vi "HFRR ADV v05 new software.vi"() -> ()   [LabVIEW 2025] (continued)
                        n2289 = property on="Humidity ( %RH )" class="WFChart (strict)"("History Data"=w3352) -> ()  [unwired: 2 in, 2 out]
                        n2290 = property on="Temperature ( Deg C )" class="WFChart (strict)"("History Data"=w3352) -> ()  [unwired: 2 in, 2 out]
                        n2291 = property on="Electrical Contact Resistance ( % )" class="WFChart (strict)"("History Data"=w3352) -> ()  [unwired: 2 in, 2 out]
                        n2292 = property on="Coefficient of Friction" class="WFChart (strict)"("History Data"=w3352) -> ()  [unwired: 2 in, 2 out]
                        n2293 = property on="Frictional Force ( N )" class="WFChart (strict)"("History Data"=w3352) -> ()  [unwired: 2 in, 2 out]
                        n2294 = property on="Coefficient of Friction" class="WFChart (strict)"("History Data"=w3352) -> ()  [unwired: 2 in, 2 out]
                        n2295 = property on="Frictional Force ( N )" class="WFChart (strict)"("History Data"=w3352) -> ()  [unwired: 2 in, 2 out]
                        n2296 = property on="Electrical Contact Resistance ( % )" class="WFChart (strict)"("History Data"=w3352) -> ()  [unwired: 2 in, 2 out]
                        n2297 = property on="Humidity ( %RH )" class="WFChart (strict)"("History Data"=w3352) -> ()  [unwired: 2 in, 2 out]
                        n2298 = property on="Stroke ( mm )" class="WFChart (strict)"("History Data"=w3353) -> ()  [unwired: 2 in, 2 out]
                        n2299 = property on="Temperature ( Deg C )" class="WFChart (strict)"("History Data"=w3352) -> ()  [unwired: 2 in, 2 out]
                        n2300 = property on="Service Password Log" class="Str"("Visible"=w3354) -> ()  [unwired: 2 in, 2 out]
                        n2301 = property on="Password 3" class="Clust (strict)"("Visible"=w3354) -> ()  [unwired: 2 in, 2 out]
                      }
                    }
                    "TEST FILE NAM,E SAVED" <- TRUE ("TEST FILE NAM,E SAVED")
                  }
                }
              }
            }
          }
        }
        n2302 = case shown="True" w2661 {
          frame False {
            n2303 = local write "tfalg"(0.0 ("tfalg")) -> ()
          }
          frame True {
            n2304 = local read "tfalg"() -> (w2806:dbl)
            n2305 = Equal?(x=w2806, y=0.0) -> (x = y?=w2807:bool)
            n2306 = case shown="True" w2807 {
              frame False {
              }
              frame True {
                n2307 = local read "Total No. of Tests"() -> (w2810:dbl)
                n2308 = local write "tfalg"(1.0 ("tfalg")) -> ()
                n2309 = local write "acq 2"(FALSE ("acq 2")) -> ()
                n2310 = Wait (ms)(milliseconds to wait=u32 200) -> ()  [unwired: 1 out]
                n2311 = Increment(x=w2810) -> (x+1=w2809:dbl)
                n2312 = local write "Total No. of Tests"(w2809) -> ()
              }
            }
          }
        }
        n2313 = local write "Test \nStatus"(w2667) -> ()
        n2314 = local write "Save"(w2667) -> ()
        n2315 = local read "Main Tab"() -> (w2624:T2)
        n2316 = case shown="True" w2648 {
          tunnel: [FALSE ("RUN") TRUE ("RUN")] -> w2647
          tunnel: [_ 1] -> w2640
          frame False {
          }
          frame True {
          }
        }
        n2317 = In Range and Coerce(upper limit=w2655, x=w2628, lower limit=w2654) -> (In Range?=w2646:bool)  [unwired: 1 out]
        n2318 = In Range and Coerce(upper limit=w2652, x=w2627, lower limit=w2653) -> (In Range?=w2644:bool)  [unwired: 1 out]
        n2319 = case shown="True" w2660 {
          frame False {
            n2320 = local read "Rt 3"() -> (w2788:bool)
            n2321 = case shown="True" w2788 {
              frame False {
              }
              frame True {
                n2322 = local write "Rt 3"(FALSE ("Rt 3")) -> ()
                n2323 = local write "Json End Flg"(TRUE ("Upld AR 2")) -> ()
              }
            }
            "Rt" <- TRUE ("Rt")
            "Rt 2" <- FALSE ("Rt")
          }
          frame True {
            n2324 = local read "Rt"() -> (w2795:bool)
            n2325 = local write "Rt 2"(TRUE ("Rt 2")) -> ()
            n2326 = case shown="True" w2795 {
              frame False {
              }
              frame True {
                w2796 = TRUE ("Upld AR 2")
                n2327 = local write "Rt"(FALSE ("Rt")) -> ()
                n2328 = local write "Upld AR"(w2796) -> ()
                n2329 = local write "Json St Flg"(w2796) -> ()
              }
            }
            "Rt 3" <- TRUE ("Rt 3")
          }
        }
        n2330 = case shown="True" w2646 {
          tunnel: [FALSE ("RUN") TRUE ("RUN")] -> w2645
          tunnel: [_ 2] -> w2639
          frame False {
          }
          frame True {
          }
        }
        n2331 = case shown="True" w2644 {
          tunnel: [FALSE ("RUN") TRUE ("RUN")] -> w2643
          tunnel: [_ 3] -> w2638
          frame False {
          }
          frame True {
          }
        }
        n2332 = case shown="\"Acquire\"" w2624 {
          tunnel: w2626 -> [_ w2857]
          frame Default {
            w2856 = 0.0 ("output")
            n2333 = local write "PID-out"(w2856) -> ()
            n2334 = local write "Frequency ( Hz )"(w2856) -> ()
          }
          frame "Acquire" {
            n2335 = stacked-sequence {
              frame #0 {
                n2336 = local read "Auto Start Test"() -> (w2861:bool)
                n2337 = case shown="True" w2861 {
                  tunnel: "RUN" -> [w2882 w2885]
                  tunnel: [w2882 w2884] -> w2862
                  frame False {
                  }
                  frame True {
                    n2338 = local read "Auto Start Temp"() -> (w2883:bool)
                    n2339 = Or(x=w2885, y=w2883) -> (x .or. y?=w2884:bool)
                  }
                }
                n2340 = local read "clk"() -> (w2881:dbl)
                n2341 = local read "Save"() -> (w2877:bool)
                n2342 = Equal?(x=w2881, y=0.0) -> (x = y?=w2878:bool)
                n2343 = And(x=w2878, y=w2877) -> (x .and. y?=w2879:bool)
                n2344 = Not(x="Engage") -> (.not. x?=w2868:bool)
                n2345 = case shown="True" w2862 {
                  tunnel: [0.0 w2905] -> w2864
                  frame False {
                    (unwired) TRUE ("Visible")
                    n2346 = local read "Auto Start Test"() -> (w2889:bool)
                    n2347 = local write "Start Time"(TRUE ("Start Time")) -> ()
                    n2348 = property on="Stroke 2" class="DigNum (strict)"("Visible"=FALSE) -> ()  [unwired: 2 in, 2 out]
                    n2349 = case shown="False" w2889 {
                      frame False {
                        n2350 = property on="Heater Button" class="Bool (strict)"("DisabledEnum"=T13."Enabled" ("Disabled")) -> ()  [unwired: 2 in, 2 out]
                        n2351 = property on="Humidity" class="Bool (strict)"("DisabledEnum"=T13."Enabled" ("Disabled")) -> ()  [unwired: 2 in, 2 out]
                      }
                      frame True {
                      }
                    }
                    n2352 = case shown="False" "TestCompFlg" {
                      frame False {
                        n2353 = local read "StartFlg"() -> (w2897:bool)
                        n2354 = case shown="True" w2897 {
                          frame False {
                          }
                          frame True {
                            n2355 = flat-sequence {
                              frame #0 {
                                n2356 = local read "EVENT LOG"() -> (w2899:string)
                                n2357 = call "Event Log.vi"("Content"="Test was interrupted", "EVENT LOG"=w2899) -> ("EVENT LOG"=w2900:string)  [unwired: 8 in, 1 out]
                                n2358 = local write "EVENT LOG"(w2900) -> ()
                              }
                              frame #1 {
                                w2901 = FALSE ("StartFlg")
                                n2359 = local write "Heater Button"(w2901) -> ()
                                n2360 = local write "StartFlg"(w2901) -> ()
                                n2361 = local write "Humidity"(w2901) -> ()
                              }
                            }
                          }
                        }
                      }
                      frame True {
                      }
                    }
                    n2362 = local write "String 14"("Test will autostart once parameters reach the set value." ("String 14")) -> ()
                  }
                  frame True {
                    (unwired) FALSE ("Visible")
                    n2363 = property on="Stroke 2" class="DigNum (strict)"("Visible"=TRUE) -> ()  [unwired: 2 in, 2 out]
                    n2364 = property on="STOP 2" class="Bool (strict)"("Disabled"=u8 2) -> ()  [unwired: 2 in, 2 out]
                    n2365 = local write "String 14"(" Running....." ("String 14")) -> ()
                    n2366 = property on="Heater Button" class="Bool (strict)"("DisabledEnum"=T13."Disabled and Grayed Out" ("Disabled")) -> ()  [unwired: 2 in, 2 out]
                    n2367 = property on="Humidity" class="Bool (strict)"("DisabledEnum"=T13."Disabled and Grayed Out" ("Disabled")) -> ()  [unwired: 2 in, 2 out]
                    n2368 = case shown="True" "Start Time" {
                      selector: "Start Time" -> [_ w2917]
                      frame False {
                      }
                      frame True {
                        n2369 = Not(x=w2917) -> (.not. x?=w2916:bool)
                        n2370 = local write "Start Time"(w2916) -> ()
                        n2371 = local read "EVENT LOG"() -> (w2918:string)
                        n2372 = call "Event Log.vi"("Content"="Test in progress", "EVENT LOG"=w2918) -> ("EVENT LOG"=w2920:string)  [unwired: 8 in, 1 out]
                        n2373 = local write "EVENT LOG"(w2920) -> ()
                      }
                    }
                    n2374 = local read "Set Hz"() -> (w2914:dbl)
                    n2375 = call <vilib>:"Uniform White Noise Waveform.vi"() -> ("signal out"=w2913:waveform(dbl))  [unwired: 10 in, 1 out]
                    n2376 = Random Number (0-1)() -> (number: 0 to 1=w2904:dbl)
                    n2377 = Add(x=w2914, y=w2913) -> (x+y=w2912:waveform(dbl))
                    n2378 = Multiply(x=ext 0.05 ("y"), y=w2904) -> (x*y=w2902:ext)
                    n2379 = Multiply(x=w2912, y=w2902) -> (x*y=w2905:waveform(ext))
                    "StartFlg" <- TRUE ("StartFlg")
                  }
                }
                n2380 = case shown="True" w2879 {
                  frame False {
                  }
                  frame True {
                    n2381 = local write "clk"(10.0 ("clk")) -> ()
                    n2382 = Get Date/Time In Seconds() -> (seconds since 1Jan1904=w2923:timestamp)
                    n2383 = To Double Precision Float(number=w2923) -> (double precision float=w2921:dbl)
                    n2384 = local write "acq timer"(w2921) -> ()
                    n2385 = local write "act save time"(w2921) -> ()
                  }
                }
                n2386 = call "Elapsed Time"("Time Target (s)"="Countdown", "Reset"=w2868) -> ("Elapsed Time (s)"=w2873:dbl, "Time has Elapsed"=w2871:bool)  [unwired: 10 in, 6 out]
                "Countdown 2" <- w2873
                n2387 = Subtract(x=w2873, y=2.0) -> (x-y=w2876:dbl)
                n2388 = Less?(x=w2876, y="Countdown") -> (x < y?=w2874:bool)
                n2389 = And(x=w2874, y=w2871) -> (x .and. y?=w2870:bool)
                n2390 = case shown="True" w2870 {
                  frame False {
                  }
                  frame True {
                    (unwired) dbl[] [] ("History Data")
                    n2391 = local write "Engage"(FALSE ("Engage")) -> ()
                    n2392 = local write "RUN"(TRUE ("RUN")) -> ()
                    n2393 = local read "Humidity ( %RH )"() -> (→"Rh Before":dbl)
                  }
                }
                n2394 = Add(x=w2864, y=50.0) -> (x+y=w2860:dbl)
                n2395 = local read "Test \nStatus"() -> (w2866:bool)
                n2396 = Select(t=w2860, s=w2866, f=0.0) -> (s? t:f=w2865:dbl)
                n2397 = local write "Frequency ( Hz )"(w2865) -> ()
              }
              frame #1 {
                w2946 = 1000000.0 ("x")
                # "HC;1/0\nST;VALUE"
                # "Elapsed time\ncof\nstroke\nAir temp\nTemp\nHumidity"
                # "acq timer\n\nact save time"
                # "convert to microseconds"
                n2398 = local read "COUNT"() -> (w2929:i32)
                n2399 = local read "Rate"() -> (w2942:dbl)
                n2400 = Divide(x=w2946, y=w2942) -> (x/y=w2947:dbl)
                n2401 = Greater Or Equal?(x=w2929, y=250) -> (x >= y?=w2928:bool)
                n2402 = Get Date/Time In Seconds() -> (seconds since 1Jan1904=w2949:timestamp)
                n2403 = case shown="True" w2928 {
                  frame False {
                    n2404 = local read "COUNT"() -> (w2950:i32)
                    n2405 = Increment(x=w2950) -> (x+1=w2951:i32)
                    n2406 = local write "COUNT"(w2951) -> ()
                  }
                  frame True {
                    n2407 = local write "COUNT"(0 ("COUNT")) -> ()
                  }
                }
                n2408 = local read "Samplingtime 2"() -> (w2927:dbl)
                n2409 = local read "act save time"() -> (w2944:dbl)
                n2410 = Divide(x=w2947, y=w2946) -> (x/y=w2945:dbl)
                n2411 = To Double Precision Float(number=w2949) -> (double precision float=w2938:dbl)
                n2412 = Add(x=w2944, y=w2927) -> (x+y=w2943:dbl)
                n2413 = local read "acq timer"() -> (w2948:dbl)
                n2414 = local read "COUNT"() -> (w2931:i32)
                n2415 = Greater Or Equal?(x=w2938, y=w2943) -> (x >= y?=w2926:bool)
                n2416 = Multiply(x=w2945, y=w2931) -> (x*y=w2937:dbl)
                n2417 = Subtract(x=w2938, y=w2948) -> (x-y=w2940:dbl)
                n2418 = local read "Save"() -> (w2941:bool)
                n2419 = Add(x=w2940, y=w2937) -> (x+y=w2924:dbl)
                "Elapsed time 3" <- w2924
                n2420 = And(x=w2926, y=w2941) -> (x .and. y?=w2939:bool)
                n2421 = Divide(x=w2924, y=60.0) -> (x/y=w2935:dbl)
                n2422 = local read "Test \nStatus"() -> (w2925:bool)
                n2423 = local read "clk"() -> (w2932:dbl)
                n2424 = Equal?(x=w2932, y=10.0) -> (x = y?=w2934:bool)
                n2425 = case shown="True" w2939 {
                  tunnel: w2938 -> [_ w3060]
                  tunnel: [FALSE ("Boolean 2") TRUE ("Boolean 2")] -> _
                  frame False {
                  }
                  frame True {
                    w3014 = ";" ("Substring")
                    # "Pid out/\nFreq response value"
                    n2426 = local write "act save time"(w3060) -> ()
                    n2427 = local read "FILE"() -> (w3008:string)
                    n2428 = call "file check.vi"("file name in"=w3008) -> ("error out"=w3011:errorcluster, "file name out"=w3006:string)  [unwired: 9 in]
                    n2429 = call "FILE PATH CREATION.vi"("error in"=w3011, "FILE NAME :"=w3006) -> ("FILE OUT"=w3009:path)  [unwired: 8 in, 1 out]
                    n2430 = Concatenate Strings(w3006, ".dgf" ("Substring")) -> (w3010:string)
                    n2431 = local read "FF 2"() -> (→"Frictional Force ( N )" →"Frictional Force ( N )":dbl)
                    n2432 = Build Path(base path=w3009, name or relative path=w3010) -> (appended path=w3005:path)
                    n2433 = local read "COF 2"() -> (w3019:dbl)
                    "cof" <- w3019
                    "Coefficient of Friction" <- w3019
                    "COF 4" <- w3019
                    "Coefficient of Friction" <- w3019
                    n2434 = local read "LVDT STROKE"() -> (w3003:dbl)
                    n2435 = local read "Add up Stroke"() -> (w3001:dbl)
                    n2436 = local read "TEMP"() -> (w3022:dbl)
                    "Temp" <- w3022
                    "Temperature ( Deg C )" <- w3022
                    n2437 = local read "Humidity ( %RH )"() -> (w3021:dbl)
                    "Humidity ( %RH )" <- w3021
                    "Humidity ( %RH )" <- w3021
                    n2438 = local read "Frequency ( Hz )"() -> (w3028:dbl)
                    n2439 = local read "Elapsed time"() -> (w3053:dbl)
                    n2440 = local read "AIR TEMP"() -> (w3026:dbl)
                    n2441 = local read "PID-out"() -> (w3031:dbl)
                    n2442 = Subtract(x=w3003, y=w3001) -> (x-y=w3002:dbl)
                    n2443 = Absolute Value(x=w3002) -> (abs(x)=w3000:dbl)
                    n2444 = local write "Temperature ( Deg C )"(w3022) -> ()
                    n2445 = Number To Fractional String(number=w3000, width (-)=i16 9 ("precision (6)"), precision (6)=i16 6) -> (F-format string=w3046:string)  [unwired: 1 in]
                    n2446 = Number To Fractional String(number=w3026, width (-)=i16 9 ("precision (6)"), precision (6)=i16 3) -> (F-format string=w3045:string)  [unwired: 1 in]
                    n2447 = Number To Fractional String(number=w3022, width (-)=i16 9 ("precision (6)"), precision (6)=i16 3) -> (F-format string=w3042:string)  [unwired: 1 in]
                    n2448 = Number To Fractional String(number=w3021, width (-)=i16 9 ("precision (6)"), precision (6)=i16 3) -> (F-format string=w3039:string)  [unwired: 1 in]
                    n2449 = Number To Fractional String(number=0.0, width (-)=i16 9 ("precision (6)"), precision (6)=i16 3) -> (F-format string=w3036:string)  [unwired: 1 in]
                    n2450 = Number To Fractional String(number=w3031, width (-)=i16 9 ("precision (6)"), precision (6)=i16 3) -> (F-format string=w3032:string)  [unwired: 1 in]
                    n2451 = Number To Fractional String(number=w3028, width (-)=i16 9 ("precision (6)"), precision (6)=i16 3) -> (F-format string=w3027:string)  [unwired: 1 in]
                    n2452 = Number To Fractional String(number=w3019, width (-)=i16 9 ("precision (6)"), precision (6)=i16 6) -> (F-format string=w3054:string)  [unwired: 1 in]
                    n2453 = Number To Fractional String(number=w3053, width (-)=i16 14 ("precision (6)"), precision (6)=i16 3) -> (F-format string=w3055:string)  [unwired: 1 in]
                    n2454 = Bundle("y"=1.02, w3000, "y"=0.98) -> (w3020:cluster{"y":dbl, dbl, "y":dbl})  [unwired: 1 in]
                    n2455 = Number To Fractional String(number="Ambient Humidity :", width (-)=i16 9 ("precision (6)"), precision (6)=i16 6) -> (F-format string=w3012:string)  [unwired: 1 in]
                    n2456 = local read "RUN"() -> (w3018:bool)
                    n2457 = case shown="True" w3018 {
                      tunnel: w3020 -> [_ w3065]
                      tunnel: w3000 -> [_ w3064]
                      tunnel: w3000 -> [_ w3062]
                      tunnel: w3000 -> [_ w3063]
                      frame False {
                      }
                      frame True {
                        "Stroke ( mm )" <- w3065
                        "Stroke ( mm )" <- w3065
                        "Stroke 4" <- w3064
                        "Stroke 3" <- w3062
                        "Stroke 2" <- w3063
                        "measured_stroke" <- w3062
                      }
                    }
                    n2458 = Concatenate Strings(w3055, w3014, w3054, w3014, w3046, w3014, w3045, w3014, w3042, w3014, w3039, w3014, w3036, w3014, w3032, w3014, w3027, w3014, w3012, "\r") -> (w3052:string)
                    n2459 = call <vilib>:"Write Characters To File.vi"("append to file? (new file:F)"=TRUE, "character string"=w3052, "file path (dialog if empty)"=w3005) -> ()  [unwired: 2 in, 1 out]
                    "refresh flag" <- TRUE ("refresh flag")
                  }
                }
                n2460 = case shown="True" w2925 {
                  tunnel: w2935 -> [_ w2961]
                  tunnel: w2940 -> [_ w2971]
                  tunnel: [0.0 w2967] -> _
                  tunnel: w2934 -> [_ w2966]
                  tunnel: [0.0 w2965] -> _
                  tunnel: w2924 -> [_ w2965]
                  tunnel: w2938 -> [w2954 _]
                  frame False {
                    n2461 = local write "acq timer"(w2954) -> ()
                    n2462 = local write "Test Duration Status"(0.0 ("Test Duration Status")) -> ()
                  }
                  frame True {
                    n2463 = local read "Set Hz"() -> (w2968:dbl)
                    n2464 = local write "Elapsed time"(w2961) -> ()
                    n2465 = local read "test time"() -> (w2960:dbl)
                    n2466 = Multiply(x=w2971, y=w2968) -> (x*y=w2970:dbl)
                    n2467 = case shown="False" w2966 {
                      tunnel: w2970 -> [w2972 _]
                      tunnel: [w2972 1.0] -> w2967
                      frame False {
                        n2468 = local write "Cycles elapsed"(w2972) -> ()
                      }
                      frame True {
                      }
                    }
                    n2469 = Greater?(x=w2961, y=w2960) -> (0:w2969:bool)
                    n2470 = Subtract(x=w2960, y=w2961) -> (x-y=w2959:dbl)
                    "time" <- w2959
                    n2471 = Multiply(x=w2959, y=60.0) -> (x*y=w2958:dbl)
                    n2472 = local write "Time Remaining"(w2958) -> ()
                    n2473 = local write "Remaining Time"(w2958) -> ()
                    n2474 = case shown="True" w2969 {
                      frame False {
                      }
                      frame True {
                        n2475 = stacked-sequence {
                          frame #0 {
                            w2975 = T13."Enabled" ("Disabled")
                            w2974 = FALSE ("TEST FILE NAM,E SAVED")
                            w2978 = "" ("FILE")
                            w2979 = TRUE ("Visible")
                            n2476 = local write "Humidity"(FALSE ("Humidity")) -> ()
                            n2477 = local write "RUN"(FALSE ("OK Button 2")) -> ()
                            n2478 = local write "Heater Button"(FALSE ("Heater Button")) -> ()
                            n2479 = local write "Auto Start Test"(FALSE ("Auto Start Test")) -> ()
                            n2480 = local write "TestCompFlg"(TRUE ("StpFlg")) -> ()
                            n2481 = local read "Humidity ( %RH )"() -> (→"Rh After":dbl)
                            n2482 = property on="STOP 2" class="Bool (strict)"("Disabled"=u8 0) -> ()  [unwired: 2 in, 2 out]
                            n2483 = local read "EVENT LOG"() -> (w2984:string)
                            n2484 = call "Event Log.vi"("Content"="Test Completed", "EVENT LOG"=w2984) -> ("EVENT LOG"=w2983:string)  [unwired: 8 in, 1 out]
                            n2485 = property on="RUN" class="Bool (strict)"("Visible"=w2979) -> ()  [unwired: 2 in, 2 out]
                            n2486 = property on="Auto Start Test" class="Bool (strict)"("Visible"=w2979) -> ()  [unwired: 2 in, 2 out]
                            n2487 = local write "Batch Ref Num :"(w2978) -> ()
                            n2488 = local write "FILE"(w2978) -> ()
                            n2489 = local write "EVENT LOG"(w2983) -> ()
                            n2490 = local write "TEST FILE NAM,E SAVED"(w2974) -> ()
                            n2491 = local write "Fuel Discription :"(w2978) -> ()
                            n2492 = local write "START TEMP"(w2974) -> ()
                            n2493 = local write "Remarks :"(w2978) -> ()
                            n2494 = local write "Main Dashboard Buttons"(T1."Imaging" ("Main Dashboard Buttons")) -> ()
                            n2495 = local write "Main Tab"(T2."Adv Scar" ("Main Tab")) -> ()
                            n2496 = property on="FRICVALZ 2" class="Bool (strict)"("DisabledEnum"=w2975) -> ()  [unwired: 2 in, 2 out]
                            n2497 = property on="FRICVALZ 3" class="Bool (strict)"("DisabledEnum"=w2975) -> ()  [unwired: 2 in, 2 out]
                            n2498 = property on="FRICVALZ 4" class="Bool (strict)"("DisabledEnum"=w2975) -> ()  [unwired: 2 in, 2 out]
                          }
                          frame #1 {
                            n2499 = Wait (ms)(milliseconds to wait=u32 1500) -> ()  [unwired: 1 out]
                          }
                          frame #2 {
                            n2500 = local write "Command"("VC;0") -> ()
                          }
                          frame #3 {
                            n2501 = Wait (ms)(milliseconds to wait=u32 1500) -> ()  [unwired: 1 out]
                          }
                          frame #4 {
                            n2502 = local write "Command"("VC;0") -> ()
                          }
                          frame #5 {
                            n2503 = Wait (ms)(milliseconds to wait=u32 1500) -> ()  [unwired: 1 out]
                          }
                          frame #6 {
                            n2504 = local write "Command"("ST;0") -> ()
                          }
                          frame #7 {
                            n2505 = local write "measured_stroke"(0.0 ("measured_stroke")) -> ()
                            n2506 = Wait (ms)(milliseconds to wait=u32 1500) -> ()  [unwired: 1 out]
                          }
                          frame #8 {
                            n2507 = local write "Command"("HE;0") -> ()
                          }
                        }
                      }
                    }
                    n2508 = Divide(x=w2961, y=w2960) -> (x/y=w2964:dbl)
                    n2509 = Multiply(x=w2964, y=100.0) -> (x*y=w2962:dbl)
                    n2510 = local write "Test Duration Status"(w2962) -> ()
                  }
                }
              }
              frame #2 {
                n2511 = case shown="True" "Heater Button" {
                  tunnel: [0.0 ("output") w3088] -> w3066
                  frame False {
                    w3069 = TRUE ("tmpchk")
                    n2512 = local read "TEMP"() -> (w3070:dbl)
                    n2513 = local write "Temp ini"(w3070) -> ()
                    n2514 = local write "Reset 4"(w3069) -> ()
                    n2515 = local write "tmpchk"(w3069) -> ()
                    n2516 = local write "reinit"(TRUE ("reinit")) -> ()
                    n2517 = local write "manual temp log"(TRUE ("manual temp log")) -> ()
                  }
                  frame True {
                    # "Logic to turn off\nthe heater when \ntemp is not rising.\nTime - 60 sec\nDelta t- 5°c"
                    n2518 = local read "Temp ini"() -> (w3077:dbl)
                    n2519 = local read "Auto Start Test"() -> (w3073:bool)
                    n2520 = Less?(x=w3077, y=53.0) -> (x < y?=w3075:bool)
                    n2521 = case shown="False" w3073 {
                      frame False {
                        n2522 = local read "Set Temp"() -> (w3097:dbl)
                        n2523 = local read "TEMP"() -> (w3096:dbl)
                        n2524 = Subtract(x=w3097, y=w3096) -> (x-y=w3095:dbl)
                        n2525 = Absolute Value(x=w3095) -> (abs(x)=w3094:dbl)
                        n2526 = Less?(x=w3094, y=0.5) -> (x < y?=w3092:bool)
                        n2527 = case shown="True" w3092 {
                          tunnel: "manual temp log" -> [_ w3098]
                          frame False {
                          }
                          frame True {
                            n2528 = case shown="True" w3098 {
                              selector: w3098 -> [_ w3099]
                              frame False {
                              }
                              frame True {
                                # "#Event log"
                                n2529 = Not(x=w3099) -> (.not. x?=w3100:bool)
                                n2530 = local write "manual temp log"(w3100) -> ()
                                n2531 = local read "EVENT LOG"() -> (w3103:string)
                                n2532 = call "Event Log.vi"("Content"="Target Temperature reached", "EVENT LOG"=w3103) -> ("EVENT LOG"=w3102:string)  [unwired: 8 in, 1 out]
                                n2533 = local write "EVENT LOG"(w3102) -> ()
                              }
                            }
                          }
                        }
                      }
                      frame True {
                        n2534 = local write "manual temp log"(TRUE ("manual temp log")) -> ()
                      }
                    }
                    n2535 = And(x="tmpchk", y=w3075) -> (x .and. y?=w3078:bool)
                    n2536 = case shown="True" w3078 {
                      frame False {
                      }
                      frame True {
                        n2537 = call "Elapsed Time8"("Time Target (s)"=300.0, "Reset"="Reset 4") -> ("Time has Elapsed"=w3105:bool)  [unwired: 10 in, 7 out]
                        n2538 = flat-sequence {
                          tunnel: w3105 -> [_]
                          frame #0 {
                            n2539 = local write "Reset 4"(FALSE ("Reset 4")) -> ()
                          }
                        }
                        n2540 = case shown="True" w3105 {
                          frame False {
                          }
                          frame True {
                            n2541 = local read "Temp ini"() -> (w3112:dbl)
                            n2542 = Add(x=w3112, y=5.0) -> (x+y=w3110:dbl)
                            n2543 = local read "TEMP"() -> (w3113:dbl)
                            n2544 = Greater?(x=w3113, y=w3110) -> (0:w3111:bool)
                            n2545 = case shown="False" w3111 {
                              frame False {
                                n2546 = local write "Heater Button"(FALSE ("Heater Button")) -> ()
                              }
                              frame True {
                                n2547 = local write "tmpchk"(FALSE ("tmpchk")) -> ()
                              }
                            }
                          }
                        }
                      }
                    }
                    n2548 = local read "Set Temp"() -> (w3086:dbl)
                    n2549 = local read "TEMP"() -> (w3080:dbl)
                    n2550 = call-poly <vilib>:"PID.vi"("reinitialize? (F)"="reinit", "dt (s)"=-1.0, "process variable"=w3080, "setpoint"=w3086) -> ("output"=w3083:dbl)  [unwired: 6 in, 1 out]
                    n2551 = Subtract(x=w3086, y=w3080) -> (x-y=w3087:dbl)
                    n2552 = Add(x=w3086, y=0.5) -> (x+y=w3084:dbl)
                    n2553 = Greater Or Equal?(x=w3080, y=w3084) -> ()  [unwired: 1 out]
                    n2554 = Select(t=0.0, s=FALSE, f=w3083) -> (s? t:f=w3082:dbl)
                    "PID output" <- w3082
                    n2555 = flat-sequence {
                      tunnel: w3082 -> [w3116]
                      tunnel: [w3116] -> w3088
                      frame #0 {
                        n2556 = local write "reinit"(FALSE ("reinit")) -> ()
                      }
                    }
                    n2557 = Bundle(w3087, "output"=w3082, "TEMP"=w3080) -> ()  [unwired: 1 in, 1 out]
                  }
                }
                "PID-out" <- w3066
              }
              frame #3 {
                n2558 = local read "TEMP"() -> (w3118:dbl)
                n2559 = Greater Or Equal?(x=w3118, y="Set Temp 2") -> (x >= y?=w3123:bool)
                n2560 = case shown="True" w3123 {
                  tunnel: [FALSE TRUE] -> w3121
                  frame False {
                  }
                  frame True {
                  }
                }
                "Status 13" <- w3121
                n2561 = And(x=w3121, y="trip1 8") -> (x .and. y?=w3120:bool)
                n2562 = case shown="True" w3120 {
                  frame False {
                    n2563 = local write "Heater Trip Temp"(TRUE ("Heater Trip Temp")) -> ()
                  }
                  frame True {
                    w3126 = FALSE ("OK Button 2")
                    n2564 = case shown="True" "Heater Trip Temp" {
                      selector: "Heater Trip Temp" -> [_ w3128]
                      frame False {
                      }
                      frame True {
                        n2565 = Not(x=w3128) -> (.not. x?=w3127:bool)
                        n2566 = local read "EVENT LOG"() -> (w3131:string)
                        n2567 = local write "Heater Trip Temp"(w3127) -> ()
                        n2568 = call "Event Log.vi"("Content"="Heater Trip", "EVENT LOG"=w3131) -> ("EVENT LOG"=w3130:string)  [unwired: 8 in, 1 out]
                        n2569 = local write "EVENT LOG"(w3130) -> ()
                      }
                    }
                    n2570 = local write "RUN"(w3126) -> ()
                    n2571 = property on="Auto Start Test" class="Bool (strict)"("Value"=w3126) -> ()  [unwired: 2 in, 2 out]
                    n2572 = local write "Heater Button"(w3126) -> ()
                  }
                }
              }
            }
            n2573 = case shown="False" w2857 {
              frame False {
                n2574 = disable-structure shown="Disabled" {
                  frame Disabled {
                    n2575 = stacked-sequence {
                      frame #0 {
                        n2576 = local write "RUN"(FALSE ("OK Button 2")) -> ()
                      }
                      frame #1 {
                      }
                    }
                  }
                  frame Enabled {
                  }
                }
              }
              frame True {
              }
            }
          }
        }
        n2577 = local read "airtempflg"() -> (w2649:bool)
        n2578 = Or(x=w2649, y=w2647) -> (x .or. y?=w2650:bool)
        n2579 = Insert Into Array(array=string[] ["Air Temperature has reached set value,", "Humidity has reached set value,", "Sample Temperaturehas reached set value,", ""], index=0, new element="") -> (w2635:string[])
        n2580 = Build Array(w2640, w2639, w2638) -> (w2636:i32[])
        n2581 = disable-structure shown="Disabled" {
          disable-tunnel: w2650 -> [w2727 _]
          disable-tunnel: w2645 -> [w2726 _]
          disable-tunnel: w2643 -> [w2725 _]
          frame Disabled {
            n2582 = Compound Arithmetic op=AND(w2727, w2726, w2725) -> ()  [unwired: 1 out]
            n2583 = case shown="True" {
              selector: _ -> [_ _]
              frame False {
              }
              frame True {
                w2728 = FALSE ("autostrtflg")
                n2584 = local write "RUN"(TRUE ("RUN")) -> ()
                n2585 = local write "autostrtflg"(w2728) -> ()
                n2586 = local write "autostart"(w2728) -> ()
                n2587 = local write "String 14"(" Running....." ("String 14")) -> ()
              }
            }
          }
          frame Enabled {
          }
        }
        n2588 = for {
          tunnel: w2636 -> [w2778] mode=indexing
          tunnel: w2635 -> [w2777]
          shift-right: [w2774] -> w2634
          shift-left: "" -> [w2776]
          n2589 = Index Array(array=w2777, index=w2778) -> (element=w2775:string)
          n2590 = Concatenate Strings(w2775, w2776) -> (w2774:string)
        }
        n2591 = local write "autostart 2"(w2634) -> ()
        n2592 = local read "Reset Graph"() -> (w2623:bool)
        n2593 = case shown="True" w2623 {
          selector: w2623 -> [_ w2677]
          frame False {
          }
          frame True {
            w2691 = 0.0 ("X Scale.Range:Maximum")
            n2594 = Not(x=w2677) -> (.not. x?=w2676:bool)
            n2595 = local write "Reset Graph"(w2676) -> ()
            n2596 = property on="Electrical Contact Resistance ( % )" class="WFChart (strict)"("XScale.Maximum"=600.0 ("X Scale.Range:Maximum"), "XScale.Minimum"=0.0 ("X Scale.Range:Minimum"), "YScale.Maximum"=100.0 ("Y Scale.Range:Maximum"), "YScale.Minimum"=0.0 ("Y Scale.Range:Minimum")) -> ()  [unwired: 2 in, 2 out]
            n2597 = property on="Frictional Force ( N )" class="WFChart (strict)"("XScale.Maximum"=600.0 ("X Scale.Range:Maximum"), "XScale.Minimum"=0.0 ("X Scale.Range:Minimum"), "YScale.Maximum"=100.0 ("Y Scale.Range:Maximum"), "YScale.Minimum"=0.0 ("Y Scale.Range:Minimum")) -> ()  [unwired: 2 in, 2 out]
            n2598 = property on="Temperature ( Deg C )" class="WFChart (strict)"("XScale.Maximum"=600.0 ("X Scale.Range:Maximum"), "XScale.Minimum"=0.0 ("X Scale.Range:Minimum"), "YScale.Maximum"=100.0 ("Y Scale.Range:Maximum"), "YScale.Minimum"=0.0 ("Y Scale.Range:Minimum")) -> ()  [unwired: 2 in, 2 out]
            n2599 = property on="Humidity ( %RH )" class="WFChart (strict)"("XScale.Maximum"=600.0 ("X Scale.Range:Maximum"), "XScale.Minimum"=0.0 ("X Scale.Range:Minimum"), "YScale.Maximum"=100.0 ("Y Scale.Range:Maximum"), "YScale.Minimum"=0.0 ("Y Scale.Range:Minimum")) -> ()  [unwired: 2 in, 2 out]
            n2600 = property on="Stroke ( mm )" class="WFChart (strict)"("XScale.Maximum"=600.0 ("X Scale.Range:Maximum"), "XScale.Minimum"=0.0 ("X Scale.Range:Minimum"), "YScale.Maximum"=100.0 ("Y Scale.Range:Maximum"), "YScale.Minimum"=0.0 ("Y Scale.Range:Minimum")) -> ()  [unwired: 2 in, 2 out]
            n2601 = property on="Coefficient of Friction" class="WFChart (strict)"("XScale.Maximum"=600.0 ("X Scale.Range:Maximum"), "XScale.Minimum"=0.0 ("X Scale.Range:Minimum"), "YScale.Maximum"=100.0 ("Y Scale.Range:Maximum"), "YScale.Minimum"=0.0 ("Y Scale.Range:Minimum")) -> ()  [unwired: 2 in, 2 out]
            n2602 = property on="Electrical Contact Resistance ( % )" class="WFChart (strict)"("XScale.Minimum"=0.0 ("X Scale.Range:Minimum"), "XScale.Maximum"=600.0 ("X Scale.Range:Maximum"), "YScale.Minimum"=0.0 ("Y Scale.Range:Minimum"), "YScale.Maximum"=100.0 ("Y Scale.Range:Maximum")) -> ()  [unwired: 2 in, 2 out]
            n2603 = property on="Temperature ( Deg C )" class="WFChart (strict)"("XScale.Minimum"=0.0 ("X Scale.Range:Minimum"), "XScale.Maximum"=600.0 ("X Scale.Range:Maximum"), "YScale.Minimum"=0.0 ("Y Scale.Range:Minimum"), "YScale.Maximum"=100.0 ("Y Scale.Range:Maximum")) -> ()  [unwired: 2 in, 2 out]
            n2604 = property on="Coefficient of Friction" class="WFChart (strict)"("XScale.Minimum"=0.0 ("X Scale.Range:Minimum"), "XScale.Maximum"=600.0 ("X Scale.Range:Maximum"), "YScale.Maximum"=1.0 ("X Scale.Range:Minimum"), "YScale.Minimum"=0.0 ("X Scale.Range:Minimum")) -> ()  [unwired: 2 in, 2 out]
            n2605 = property on="Frictional Force ( N )" class="WFChart (strict)"("XScale.Maximum"=600.0 ("X Scale.Range:Maximum"), "XScale.Minimum"=w2691, "YScale.Maximum"=10.0 ("Y Scale.Range:Maximum"), "YScale.Minimum"=w2691) -> ()  [unwired: 2 in, 2 out]
            n2606 = property on="Stroke ( mm )" class="WFChart (strict)"("XScale.Maximum"=600.0 ("X Scale.Range:Maximum"), "XScale.Minimum"=0.0 ("X Scale.Range:Minimum"), "YScale.Maximum"=100.0 ("Y Scale.Range:Maximum"), "YScale.Minimum"=0.0 ("Y Scale.Range:Minimum")) -> ()  [unwired: 2 in, 2 out]
            n2607 = property on="Humidity ( %RH )" class="WFChart (strict)"("XScale.Maximum"=600.0 ("X Scale.Range:Maximum"), "XScale.Minimum"=0.0 ("X Scale.Range:Minimum"), "YScale.Maximum"=100.0 ("Y Scale.Range:Maximum"), "YScale.Minimum"=0.0 ("Y Scale.Range:Minimum")) -> ()  [unwired: 2 in, 2 out]
          }
        }
      }
      frame "Compare Files" {
        # "Elapsed time\ncof\nstroke\nAir temp\nTemp\nHumidity"
        n2608 = case shown="True" "RSTV1 2" {
          frame False {
          }
          frame True {
            n2609 = property on="Humidity ( %RH )" class="XYGraph (strict)"("Y Scale.Display Format:Precision"=u8 0 ("Y Scale.Format & Precision:Precision")) -> ()  [unwired: 2 in, 2 out]
            n2610 = property on="Humidity ( %RH )" class="XYGraph (strict)"("X Scale.Range:Minimum"=0.0, "X Scale.Range:Maximum"=75.0, "Y Scale.Range:Minimum"=48.0, "Y Scale.Range:Maximum"=58.0) -> ()  [unwired: 2 in, 2 out]
          }
        }
        n2611 = case shown="True" "RST CP 2" {
          frame False {
          }
          frame True {
            n2612 = property on="XY Graph 13" class="XYGraph (strict)"("Y Scale.Display Format:Precision"=u8 0 ("Y Scale.Format & Precision:Precision")) -> ()  [unwired: 2 in, 2 out]
            n2613 = property on="XY Graph 13" class="XYGraph (strict)"("X Scale.Range:Minimum"=0.0, "X Scale.Range:Maximum"=75.0, "Y Scale.Range:Minimum"=0.0, "Y Scale.Range:Maximum"=100.0) -> ()  [unwired: 2 in, 2 out]
          }
        }
        n2614 = case shown="True" "RST CP" {
          frame False {
          }
          frame True {
            n2615 = property on="Sample Temperature ( °C )" class="XYGraph (strict)"("Y Scale.Display Format:Precision"=u8 2 ("Y Scale.Format & Precision:Precision")) -> ()  [unwired: 2 in, 2 out]
            n2616 = property on="Sample Temperature ( °C )" class="XYGraph (strict)"("X Scale.Range:Minimum"=0.0, "X Scale.Range:Maximum"=75.0, "Y Scale.Range:Minimum"=58.0, "Y Scale.Range:Maximum"=62.0) -> ()  [unwired: 2 in, 2 out]
          }
        }
        n2617 = case shown="True" "RSTV1 3" {
          frame False {
          }
          frame True {
            n2618 = property on="Air Temperature  ( °C )" class="XYGraph (strict)"("Y Scale.Display Format:Precision"=u8 2 ("Y Scale.Format & Precision:Precision")) -> ()  [unwired: 2 in, 2 out]
            n2619 = property on="Air Temperature  ( °C )" class="XYGraph (strict)"("X Scale.Range:Minimum"=0.0 ("Y Scale.Range:Minimum"), "X Scale.Range:Maximum"=75.0 ("Y Scale.Range:Maximum"), "Y Scale.Range:Minimum"=20.0 ("X Scale.Range:Minimum"), "Y Scale.Range:Maximum"=26.0 ("X Scale.Range:Maximum")) -> ()  [unwired: 2 in, 2 out]
          }
        }
        n2620 = case shown="True" "RSTV1 4" {
          frame False {
          }
          frame True {
            n2621 = property on="Stroke ( mm )" class="XYGraph (strict)"("Y Scale.Display Format:Precision"=u8 2 ("Y Scale.Format & Precision:Precision")) -> ()  [unwired: 2 in, 2 out]
            n2622 = property on="Stroke ( mm )" class="XYGraph (strict)"("X Scale.Range:Minimum"=0.0 ("Y Scale.Range:Maximum"), "X Scale.Range:Maximum"=75.0 ("X Scale.Range:Minimum"), "Y Scale.Range:Minimum"=0.98, "Y Scale.Range:Maximum"=1.02) -> ()  [unwired: 2 in, 2 out]
          }
        }
        n2623 = case shown="True" "rstv2" {
          frame False {
          }
          frame True {
            n2624 = property on="Coefficient Of Friction" class="XYGraph (strict)"("Y Scale.Display Format:Precision"=u8 3 ("Y Scale.Format & Precision:Precision")) -> ()  [unwired: 2 in, 2 out]
            n2625 = property on="Coefficient Of Friction" class="XYGraph (strict)"("X Scale.Range:Minimum"=0.0 ("Y Scale.Range:Maximum"), "X Scale.Range:Maximum"=75.0, "Y Scale.Range:Minimum"=0.0, "Y Scale.Range:Maximum"=1.0 ("X Scale.Range:Minimum")) -> ()  [unwired: 2 in, 2 out]
          }
        }
        n2626 = case shown="True" "RST CP 3" {
          frame False {
          }
          frame True {
            n2627 = property on="Air Temp ( °C ) vs Humidity ( % RH )" class="XYGraph (strict)"("X Scale.Range:Minimum"=18.0, "X Scale.Range:Maximum"=28.0 ("X Scale.Range:Minimum"), "Y Scale.Range:Minimum"=30.0 ("X Scale.Range:Minimum"), "Y Scale.Range:Maximum"=70.0 ("X Scale.Range:Minimum")) -> ()  [unwired: 2 in, 2 out]
          }
        }
        n2628 = case shown="True" "OPEN 1" {
          frame False {
          }
          frame True {
            (unwired) 0  # existing file
            w3407 = "Choose a datalog file to open"  # prompt
            n2629 = local write "OPEN 1"(FALSE ("OPEN 1")) -> ()
            n2630 = String To Path(string="C:\\LAB-IQ\\Data\\") -> (path=w3392:path)
            n2631 = File Dialog(6:"*.dgf" ("pattern"), 7:w3407, 11:w3392) -> (0:w3390:errorcluster, 3:w3398:path)  [unwired: 4 in, 2 out]
            n2632 = Unbundle(w3390) -> ()  [unwired: 3 out]
            n2633 = Strip Path(path=w3398) -> (name=w3397:string)  [unwired: 1 out]
            n2634 = Path To String(path=w3398) -> (string=w3393:string)
            "string1" <- w3393
            n2635 = Match Pattern(string=w3397, regular expression=".dgf") -> (before substring=→"String Control":string)  [unwired: 1 in, 3 out]
            n2636 = Match Pattern(string=w3393, regular expression=".dgf" ("substring (\"\")")) -> (before substring=w3403:string)  [unwired: 1 in, 3 out]
            n2637 = Concatenate Strings(w3403, ".duf" ("Substring")) -> (w3399:string)
            n2638 = String To Path(string=w3399) -> (path=w3404:path)
            n2639 = call <vilib>:"Read Characters From File.vi"("file path (dialog if empty)"=w3404, "start of read offset (chars.:0)"=60 ("start of read offset (chars.: 0)")) -> ("character string"=→"String Control 2":string)  [unwired: 4 in, 3 out]
          }
        }
        n2640 = case shown="True" "OPEN 2" {
          frame False {
          }
          frame True {
            (unwired) 0  # existing file
            w3425 = "Choose a datalog file to open"  # prompt
            n2641 = local write "OPEN 2"(FALSE ("OPEN 1")) -> ()
            n2642 = String To Path(string="C:\\LAB-IQ\\Data\\") -> (path=w3410:path)
            n2643 = File Dialog(6:"*.dgf" ("pattern"), 7:w3425, 11:w3410) -> (0:w3408:errorcluster, 3:w3416:path)  [unwired: 4 in, 2 out]
            n2644 = Unbundle(w3408) -> ()  [unwired: 3 out]
            n2645 = Strip Path(path=w3416) -> (name=w3414:string)  [unwired: 1 out]
            n2646 = Path To String(path=w3416) -> (string=w3411:string)
            "string1 2" <- w3411
            n2647 = Match Pattern(string=w3414, regular expression=".dgf") -> (before substring=→"String Control 3":string)  [unwired: 1 in, 3 out]
            n2648 = Match Pattern(string=w3411, regular expression=".dgf" ("substring (\"\")")) -> (before substring=w3422:string)  [unwired: 1 in, 3 out]
            n2649 = Concatenate Strings(w3422, ".duf" ("Substring")) -> (w3419:string)
            n2650 = String To Path(string=w3419) -> (path=w3417:path)
            n2651 = call <vilib>:"Read Characters From File.vi"("file path (dialog if empty)"=w3417, "start of read offset (chars.:0)"=60 ("start of read offset (chars.: 0)")) -> ("character string"=→"String Control 4":string)  [unwired: 4 in, 3 out]
          }
        }
        n2652 = case shown="True" "OPEN 3" {
          frame False {
          }
          frame True {
            (unwired) 0  # existing file
            w3443 = "Choose a datalog file to open"  # prompt
            n2653 = local write "OPEN 3"(FALSE ("OPEN 1")) -> ()
            n2654 = String To Path(string="C:\\LAB-IQ\\Data\\") -> (path=w3428:path)
            n2655 = File Dialog(6:"*.dgf" ("pattern"), 7:w3443, 11:w3428) -> (0:w3426:errorcluster, 3:w3434:path)  [unwired: 4 in, 2 out]
            n2656 = Unbundle(w3426) -> ()  [unwired: 3 out]
            n2657 = Strip Path(path=w3434) -> (name=w3432:string)  [unwired: 1 out]
            n2658 = Path To String(path=w3434) -> (string=w3429:string)
            "string1 3" <- w3429
            n2659 = Match Pattern(string=w3432, regular expression=".dgf") -> (before substring=→"String Control 5":string)  [unwired: 1 in, 3 out]
            n2660 = Match Pattern(string=w3429, regular expression=".dgf" ("substring (\"\")")) -> (before substring=w3439:string)  [unwired: 1 in, 3 out]
            n2661 = Concatenate Strings(w3439, ".duf" ("Substring")) -> (w3436:string)
            n2662 = String To Path(string=w3436) -> (path=w3440:path)
            n2663 = call <vilib>:"Read Characters From File.vi"("file path (dialog if empty)"=w3440, "start of read offset (chars.:0)"=60 ("start of read offset (chars.: 0)")) -> ("character string"=→"String Control 6":string)  [unwired: 4 in, 3 out]
          }
        }
        n2664 = case shown="True" "OPEN 4" {
          frame False {
          }
          frame True {
            (unwired) 0  # existing file
            w3461 = "Choose a datalog file to open"  # prompt
            n2665 = local write "OPEN 4"(FALSE ("OPEN 1")) -> ()
            n2666 = String To Path(string="C:\\LAB-IQ\\Data\\") -> (path=w3446:path)
            n2667 = File Dialog(6:"*.dgf" ("pattern"), 7:w3461, 11:w3446) -> (0:w3444:errorcluster, 3:w3452:path)  [unwired: 4 in, 2 out]
            n2668 = Unbundle(w3444) -> ()  [unwired: 3 out]
            n2669 = Strip Path(path=w3452) -> (name=w3450:string)  [unwired: 1 out]
            n2670 = Path To String(path=w3452) -> (string=w3447:string)
            "string1 4" <- w3447
            n2671 = Match Pattern(string=w3450, regular expression=".dgf") -> (before substring=→"String Control 7":string)  [unwired: 1 in, 3 out]
            n2672 = Match Pattern(string=w3447, regular expression=".dgf" ("substring (\"\")")) -> (before substring=w3457:string)  [unwired: 1 in, 3 out]
            n2673 = Concatenate Strings(w3457, ".duf" ("Substring")) -> (w3454:string)
            n2674 = String To Path(string=w3454) -> (path=w3458:path)
            n2675 = call <vilib>:"Read Characters From File.vi"("file path (dialog if empty)"=w3458, "start of read offset (chars.:0)"=60 ("start of read offset (chars.: 0)")) -> ("character string"=→"String Control 8":string)  [unwired: 4 in, 3 out]
          }
        }
      }
      frame "About" {
        # "Elapsed time\ncof\nstroke\nmean pos\nTemp\nHumidity"
        n2676 = disable-structure shown="Disabled" {
          frame Disabled {
            n2677 = case shown="True" "Export" {
              frame False {
              }
              frame True {
                w3483 = "                                      " ("string")
                w3485 = "\r"
                (unwired) i16 6 ("width (-)")
                w3562 = "\r"
                w3494 = "\r"
                n2678 = local write "Export"(FALSE ("Export")) -> ()
                n2679 = local read "String 29"() -> (w3531:string)
                n2680 = local read "String 34"() -> (w3519:string)
                n2681 = local read "String 35"() -> (w3514:string)
                n2682 = local read "String 37"() -> (w3510:string)
                n2683 = local read "String 36"() -> (w3507:string)
                n2684 = local read "String 38"() -> (w3504:string)
                n2685 = local read "String 39"() -> (w3501:string)
                n2686 = Match Pattern(string=w3531, regular expression=".dwm") -> (before substring=w3527:string)  [unwired: 1 in, 3 out]
                "before substring" <- w3527
                n2687 = local read "S 38"() -> (w3522:string)
                n2688 = local read "S 39"() -> (w3515:string)
                n2689 = local read "Temperature before test 2"() -> (w3551:dbl)
                n2690 = local read "Temperature after test 2"() -> (w3556:dbl)
                n2691 = local read "Humidity before test 2"() -> (w3537:dbl)
                n2692 = local read "Humidity after test 2"() -> (w3552:dbl)
                n2693 = local read "MWSD 2"() -> (w3548:dbl)
                n2694 = local read "WS1.4 2"() -> (w3564:dbl)
                n2695 = local read "HCF 2"() -> (w3560:dbl)
                n2696 = local read "AVP 2"() -> (w3549:dbl)
                n2697 = Concatenate Strings("1," ("string"), w3522) -> (w3521:string)
                n2698 = Concatenate Strings("2," ("string"), w3519) -> (w3518:string)
                n2699 = Concatenate Strings("3," ("string"), w3515) -> (w3517:string)
                n2700 = Concatenate Strings("4," ("string"), w3514) -> (w3513:string)
                n2701 = Concatenate Strings("5," ("string"), w3510) -> (w3511:string)
                n2702 = Concatenate Strings("6," ("string"), w3507) -> (w3508:string)
                n2703 = Concatenate Strings("7," ("string"), w3504) -> (w3505:string)
                n2704 = Concatenate Strings("8," ("string"), w3501) -> (w3502:string)
                n2705 = local read "Sample ID"() -> (w3569:string)
                n2706 = case shown="\"xlx\"" "Select File Type" {
                  tunnel: w3527 -> [w3572 w3574 w3576]
                  tunnel: [w3570 w3575 w3577] -> w3526
                  frame "xlx" {
                    n2707 = Concatenate Strings(w3572, ".xls" ("string")) -> (w3570:string)
                  }
                  frame "csv" {
                    n2708 = Concatenate Strings(w3574, ".csv" ("string")) -> (w3575:string)
                  }
                  frame "txt" {
                    n2709 = Concatenate Strings(w3576, ".txt" ("string")) -> (w3577:string)
                  }
                }
                n2710 = local read "Test Date"() -> (w3568:string)
                n2711 = local read "String 45"() -> (w3482:string)
                n2712 = local read "String 31"() -> (w3567:string)
                n2713 = local read "String 32"() -> (w3566:string)
                n2714 = local read "TITTLE"() -> (w3490:string)
                n2715 = Number To Fractional String(number=w3537, width (-)=i16 6, precision (6)=i16 2) -> (F-format string=w3536:string)  [unwired: 1 in]
                n2716 = Number To Fractional String(number=w3551, width (-)=i16 6, precision (6)=i16 2) -> (F-format string=w3557:string)  [unwired: 1 in]
                n2717 = Number To Fractional String(number=w3552, width (-)=i16 6, precision (6)=i16 2) -> (F-format string=w3550:string)  [unwired: 1 in]
                n2718 = Number To Fractional String(number=w3556, width (-)=i16 6, precision (6)=i16 2) -> (F-format string=w3555:string)  [unwired: 1 in]
                n2719 = Number To Fractional String(number=w3548, width (-)=i16 6, precision (6)=i16 2) -> (F-format string=w3546:string)  [unwired: 1 in]
                n2720 = Number To Fractional String(number=w3549, width (-)=i16 6, precision (6)=i16 2) -> (F-format string=w3547:string)  [unwired: 1 in]
                n2721 = Number To Fractional String(number=w3560, width (-)=i16 6, precision (6)=i16 2) -> (F-format string=w3561:string)  [unwired: 1 in]
                n2722 = Number To Fractional String(number=w3564, precision (6)=i16 2) -> (F-format string=w3565:string)  [unwired: 2 in]
                n2723 = local read "s.NO"() -> (w3484:string)
                n2724 = Concatenate Strings("=" ("string"), w3490) -> (w3489:string)
                n2725 = Concatenate Strings("S.No," ("string"), "                                       Parameters" ("string")) -> (w3495:string)
                n2726 = Concatenate Strings(w3562, w3521, w3536, w3562, w3518, w3557, w3562, w3517, w3550, w3562, w3513, w3555, w3562, w3511, w3546, w3562, w3508, w3547, w3562, w3505, w3561, w3562, w3502, w3565) -> (w3524:string)
                n2727 = Concatenate Strings(w3494, "," ("string"), w3482, w3484, w3483, w3566, w3569, w3483, w3567, w3568, w3494) -> (w3492:string)
                n2728 = local read "Tested by"() -> (w3498:string)
                n2729 = local read "String 33"() -> (w3499:string)
                n2730 = Concatenate Strings("," ("string"), "                                                                             " ("string")) -> (w3487:string)
                n2731 = Concatenate Strings(w3489, w3485, w3492, w3485, w3495, w3524, w3485, w3487, w3499, w3498) -> (→"export":string)
                n2732 = String To Path(string=w3526) -> (path=w3533:path)
                n2733 = local read "export"() -> (w3528:string)
                n2734 = call <vilib>:"Write Characters To File.vi"("append to file? (new file:F)"=FALSE, "character string"=w3528, "file path (dialog if empty)"=w3533) -> ()  [unwired: 2 in, 1 out]
              }
            }
          }
          frame Enabled {
          }
        }
